vi "default setpoint.vi"(0 "error in (no error)":errorcluster, 7 "Def Set":dbl=50.0 caption="Default Setpoint (C)" format="%.2f") -> (4 "error out":errorcluster)   [LabVIEW 2016]
doc: "This vi sets the default set point\n\nerror feedthrough for wiring convenience\n\nPaul K Dixon\nPhysics 350\nCSUSB Physics"
uses:
  temp control/globals/temp control global variables.vi
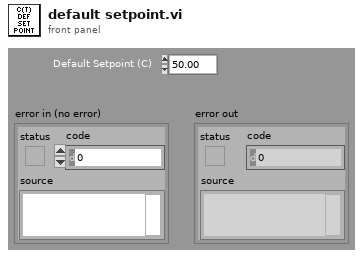
[diagram p1: front panel]
types:
  T1 = typedef "control parameters.ctl" = cluster{"Setpoint":dbl, "Control bandwidth":dbl, "Settle bandwidth":dbl, "Integral time":dbl, "Int\non":bool, "Derivative time":dbl, "Der\non":bool, "Settle time":dbl}
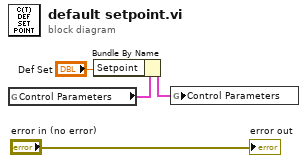
[diagram p0: block diagram]
diagram:
  n1 = global read "temp control global variables.vi" "Control Parameters"() -> (w3:T1)
  n2 = Bundle By Name(cluster=w3, "Setpoint"="Def Set") -> (w2:T1)
  n3 = global write "temp control global variables.vi" "Control Parameters"(w2) -> ()
  "error out" <- "error in (no error)"
